vi "Dig.vi"(8 "Error In":errorcluster) -> (0 "Error Out":errorcluster)   [LabVIEW 2018, in "Tests.lvlib" / "Toolkit.lvlib"]
uses:
  Toolkit.lvlib
  src/Toolkit/Toolkit.lvlib
  <vilib>/addons/_JKI Toolkits/Caraya/classes/Test/Test.lvclass
  <vilib>/addons/_JKI Toolkits/Caraya/classes/Assert/Assert.lvclass
  Tests.lvlib
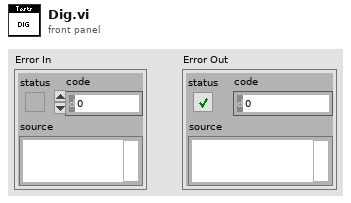
[diagram p1: front panel]
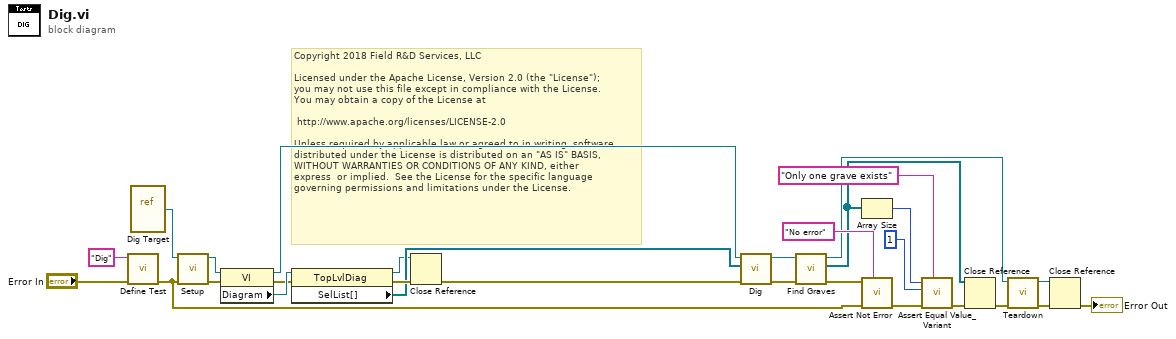
[diagram p0: block diagram]
diagram:
  # "Copyright 2018 Field R&D Services, LLC\n\nLicensed under the Apache License, Version 2.0 (the \"License\");\nyou may not use this file except in compliance with the License.\nYou may obtain a copy of the License at\n\n\thttp://www.apache.org/licenses/LICENSE-2.0\n\nUnless required by applicable law or agreed to in writing, software\ndistributed under the License is distributed on an \"AS IS\" BASIS,\nWITHOUT WARRANTIES OR CONDITIONS OF ANY KIND, either \nexpress  or implied.  See the License for the specific language \ngoverning permissions and limitations under the License."
  n1 = call <vilib>:"Define Test.vi"("error in (no error)"="Error In", "Label (VI Title)"="Dig") -> ("error out"=w6:errorcluster)  [unwired: 9 in]
  n2 = vi-ref "Dig Target.vi"() -> (w25:refnum<vi>)
  n3 = call "Setup.vi"("Error In"=w6, "VI In"=w25) -> ("Error Out"=w5:errorcluster, "VI Out"=w7:refnum<vi>)  [unwired: 8 in]
  n4 = property class="VI"(reference=w7, error in=w5) -> (reference out=w24:refnum<vi>, error out=w27:errorcluster, "Diagram"=w28:refnum<vi>)
  n5 = property class="TopLvlDiag"(reference=w28, error in=w27) -> (reference out=w15:refnum<vi>, error out=w26:errorcluster, "SelList[]"=w23:refnum<vi>[])
  n6 = Close Reference(reference=w15, error in (no error)=w26) -> (error out=w16:errorcluster)
  n7 = call "Dig.vi"("Error In"=w16, "Selection List[]"=w23, "VI In"=w24) -> ("Error Out"=w22:errorcluster, "VI Out"=w1:refnum<vi>)  [unwired: 7 in]
  n8 = call "Find Graves.vi"("Error In"=w22, "VI In"=w1) -> ("Error Out"=w17:errorcluster, "Graves"=w8:refnum<vi>[], "VI Out"=w10:refnum<vi>)  [unwired: 7 in]
  n9 = Array Size(array=w8) -> (size(s)=w14:i32)
  n10 = call <vilib>:"Assert Not Error.vi"("Label"="No error", "error in (no error)"=w6, "Not Error?"=w17) -> ("error out"=w19:errorcluster)  [unwired: 8 in]
  n11 = call <vilib>:"Assert Equal Value_Variant.vi"("Label"="Only one grave exists", "error in (no error)"=w19, "Y"=1 ("size(s)"), "X"=w14) -> ("error out"=w11:errorcluster)  [unwired: 7 in]
  n12 = Close Reference(reference=w8, error in (no error)=w11) -> (error out=w3:errorcluster)
  n13 = call "Teardown.vi"("Error In"=w3, "VI In"=w10) -> ("Error Out"=w2:errorcluster, "VI Out"=w4:refnum<vi>)  [unwired: 8 in]
  n14 = Close Reference(reference=w4, error in (no error)=w2) -> (error out=→"Error Out":errorcluster)
